vi "数组与簇互换函数.vi"() -> ()   [LabVIEW 2013]
panel:
  out "反转后的簇":T1
  in  "簇":T2
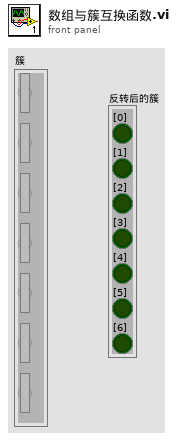
[diagram p1: front panel]
types:
  T1 = cluster{"[0]":bool, "[1]":bool, "[2]":bool, "[3]":bool, "[4]":bool, "[5]":bool, "[6]":bool}
  T2 = cluster{"布尔":bool, "布尔 2":bool, "布尔 3":bool, "布尔 4":bool, "布尔 5":bool, "布尔 6":bool, "布尔 7":bool}
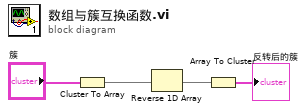
[diagram p0: block diagram]
diagram:
  n1 = Cluster To Array(cluster="簇") -> (array=w2:bool[])
  n2 = Reverse 1D Array(array=w2) -> (reversed array=w3:bool[])
  n3 = Array To Cluster(array=w3) -> (cluster=→"反转后的簇":T1)
